vi "FindTesterVI.vi"(7 "Module Name":string, 8 "error in (no error)":errorcluster, 11 "module ref":refnum<vi>) -> (0 "error out":errorcluster, 3 "TesterPath":path)   [LabVIEW 2024]
panel:
  out "Check":bool
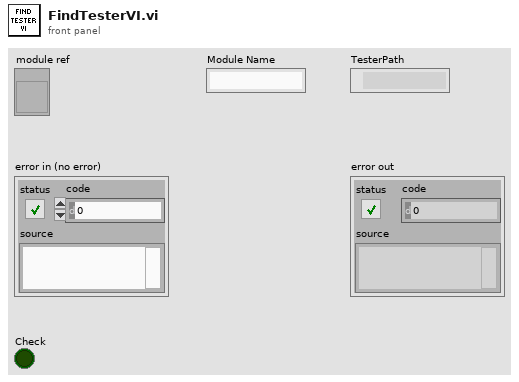
[diagram p1: front panel]
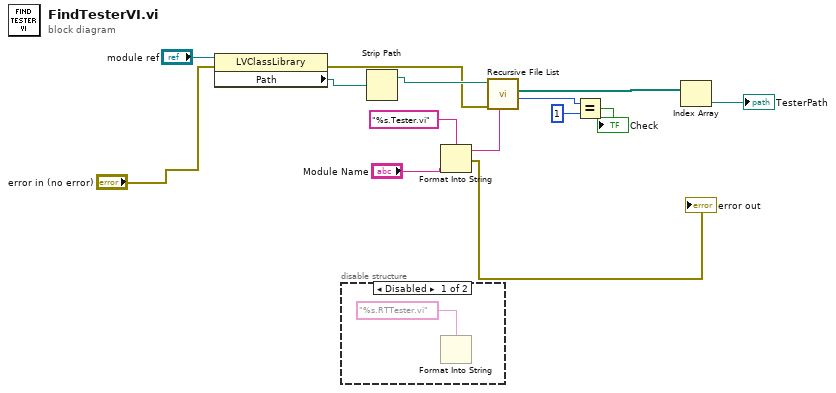
[diagram p0: block diagram]
diagram:
  n1 = property class="LVClassLibrary"(reference="module ref", error in="error in (no error)") -> (error out=w4:errorcluster, "Path"=w13:path)  [unwired: 1 out]
  n2 = disable-structure shown="Disabled" {
    frame Disabled {
      n3 = Format Into String(format string="%s.RTTester.vi" ("pattern")) -> ()  [unwired: 3 in, 2 out]
    }
    frame Enabled {
    }
  }
  n4 = Strip Path(path=w13) -> (stripped path=w12:path)  [unwired: 1 out]
  n5 = Format Into String(format string="%s.Tester.vi" ("pattern"), "Module Name") -> (resulting string=w10:string, error out=→"error out":errorcluster)  [unwired: 2 in]
  n6 = call <vilib>:"Recursive File List.vi"("pattern"=w10, "error in (no error)"=w4, "Folder Path"=w12) -> ("Number of Files"=w9:i32, "All Files in Dir"=w7:path[])  [unwired: 4 in, 3 out]
  n7 = Equal?(x=w9, y=1) -> (x = y?=→"Check":bool)
  n8 = Index Array(array=w7) -> (element=→"TesterPath":path)  [unwired: 1 in]
